vi "Get Instrument Type ID.vi"(8 "error in (no error)":errorcluster, 11 "instrument in":refnum<class "Instrument.lvclass">) -> (0 "error out":errorcluster, 2 "instrument type id":string, 3 "instrument out":refnum<class "Instrument.lvclass">)   [LabVIEW 2020, in "MeasurementLink niDCPower.lvlib" / "Instrument.lvclass"]
doc: "Returns the type ID for the instrument in the pin map file. When using third party instruments not natively supported by the pin map editor, you must create a custom instrument in the pin map file and assign it a unique instrument type ID. Return the same instrument type ID from this method to access the third party instrument from within MeasurementLink."
uses:
  Instrument.lvclass
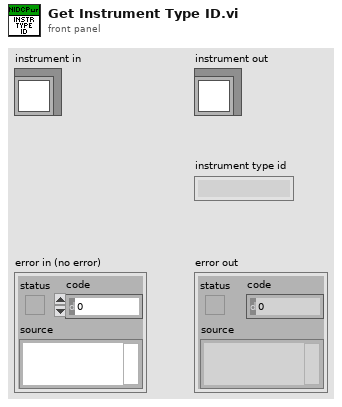
[diagram p1: front panel]
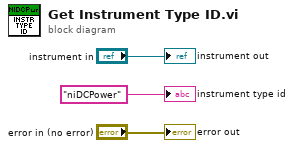
[diagram p0: block diagram]
diagram:
  "error out" <- "error in (no error)"
  "instrument out" <- "instrument in"
  "instrument type id" <- "niDCPower" ("instrument type id")
